vi "SimulateCore.vi"(8 "error in (no error)":errorcluster, 9 "Payload":string, 10 "Command":string, 11 "MicronGRPCClient in":refnum<class "MicronGRPCClient.lvclass">) -> (0 "error out":errorcluster, 2 "Response":string, 3 "MicronGRPCClient out":refnum<class "MicronGRPCClient.lvclass">)   [LabVIEW 2019, in "MicronGRPCClient.lvclass"]
uses:
  MicronGRPCClient.lvclass
  Base/Client/MicronClient.lvclass
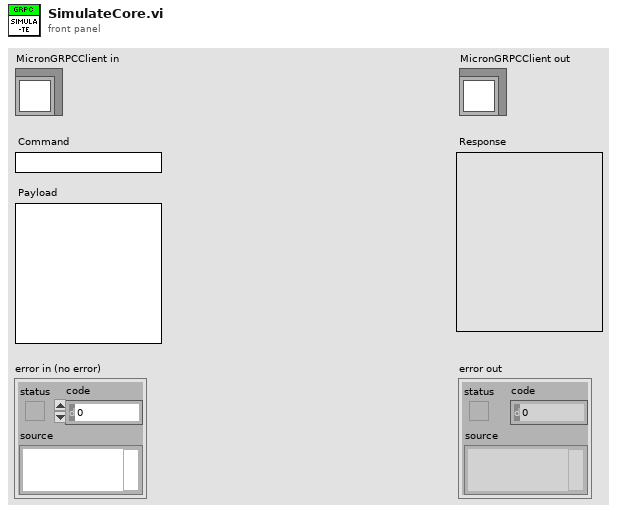
[diagram p1: front panel]
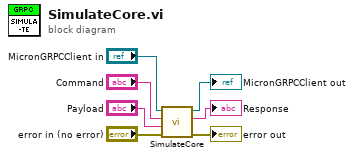
[diagram p0: block diagram]
diagram:
  n1 = call-parent "SimulateCore.vi"("error in (no error)"="error in (no error)", "Payload"="Payload", "Command"="Command", "MicronClient in"="MicronGRPCClient in") -> ("error out"=→"error out":errorcluster, "Response"=→"Response":string, "MicronClient out"=→"MicronGRPCClient out":refnum<class "MicronGRPCClient.lvclass">)  [unwired: 5 in]
